vi "video.create.vi"(8 "error in":errorcluster, 11 "Client in":refnum<class "Client.lvclass">) -> (0 "error out":errorcluster, 3 "Client out":refnum<class "Client.lvclass">)   [LabVIEW 2020, in "Client.lvclass"]
doc: "Creates a new empty video (metadata shell) with a name and optional description in Nominal and returns a handle to it."
uses:
  Client.lvclass
  client.lvlib
panel:
  out "out_video out":i32
  in  "name":string
  in  "description":string
  in  "out_video":i32
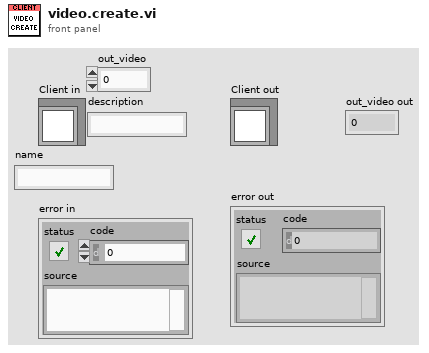
[diagram p1: front panel]
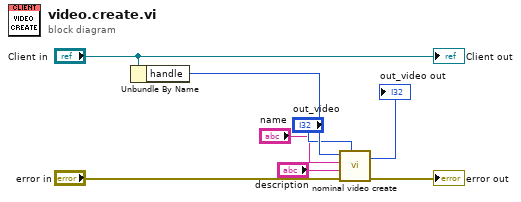
[diagram p0: block diagram]
diagram:
  n1 = Unbundle By Name("Client in") -> ("handle"=w6:i32)
  n2 = call "nominal video create.vi"("out_video"="out_video", "error in (no error)"="error in", "description"="description", "name"="name", "client"=w6) -> ("error out"=→"error out":errorcluster, "out_video out"=→"out_video out":i32)  [unwired: 4 in, 1 out]
  "Client out" <- "Client in"
